vi "Eventos.vi"() -> ()   [LabVIEW 2018]
uses:
  <vilib>/RAFA Solutions/Harmony UI Controls Kit/String & Path/String Indicator.ctl
  <vilib>/RAFA Solutions/Harmony UI Controls Kit/Boolean/OK Button.ctl
  <vilib>/RAFA Solutions/Harmony UI Controls Kit/Boolean/Blank Button - Green.ctl
  Controls/Hora y Fecha control.ctl
  <vilib>/RAFA Solutions/Harmony UI Controls Kit/List, Table & Tree/Multicolumn Listbox.ctl
  <vilib>/RAFA Solutions/Harmony UI Controls Kit/Flat UI Design.lvlib
panel:
  in  "Tabla Eventos":T1
  out "fecha y hora":T2
  in  "Tiempo Final Eventos":timestamp caption="Tiempo Final" format="%<%X\n%x>T"
  in  "Tiempo Inicio Eventos":timestamp caption="Tiempo Inicio" format="%<%X\n%x>T"
  in  "Consultar Eventos":T3
  out "Generador":string
  in  "volver":T4
  out "Eventos":T5
  # "Sistema de Monitoreo de Calidad de Energía"
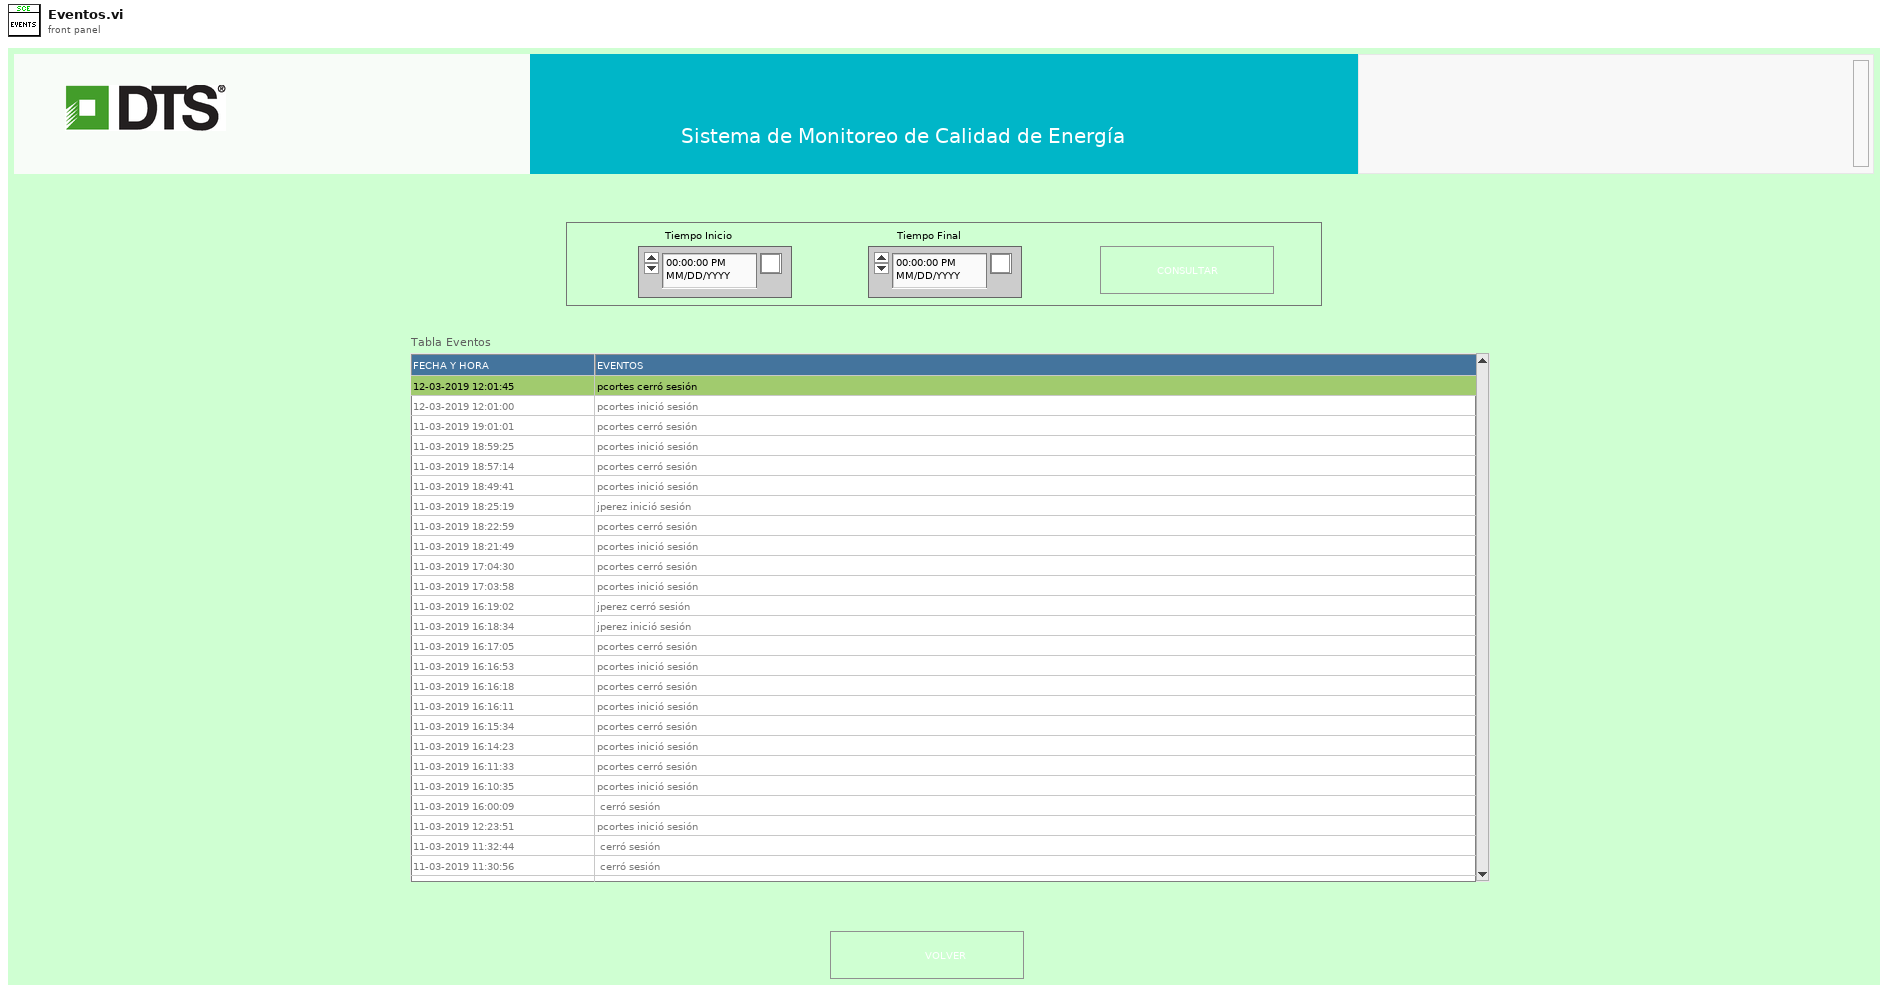
[diagram p1: front panel]
types:
  T1 = typedef "Flat UI Design.lvlib/Multicolumn Listbox.ctl" = i32
  T2 = typedef "Hora y Fecha control.ctl" = cluster{"fecha":string, "dia semana":string, "fecha 2":string}
  T3 = typedef "Flat UI Design.lvlib/Blank Button - Green.ctl" = bool
  T4 = typedef "Flat UI Design.lvlib/OK Button.ctl" = bool
  T5 = typedef "Flat UI Design.lvlib/String Indicator.ctl" = string
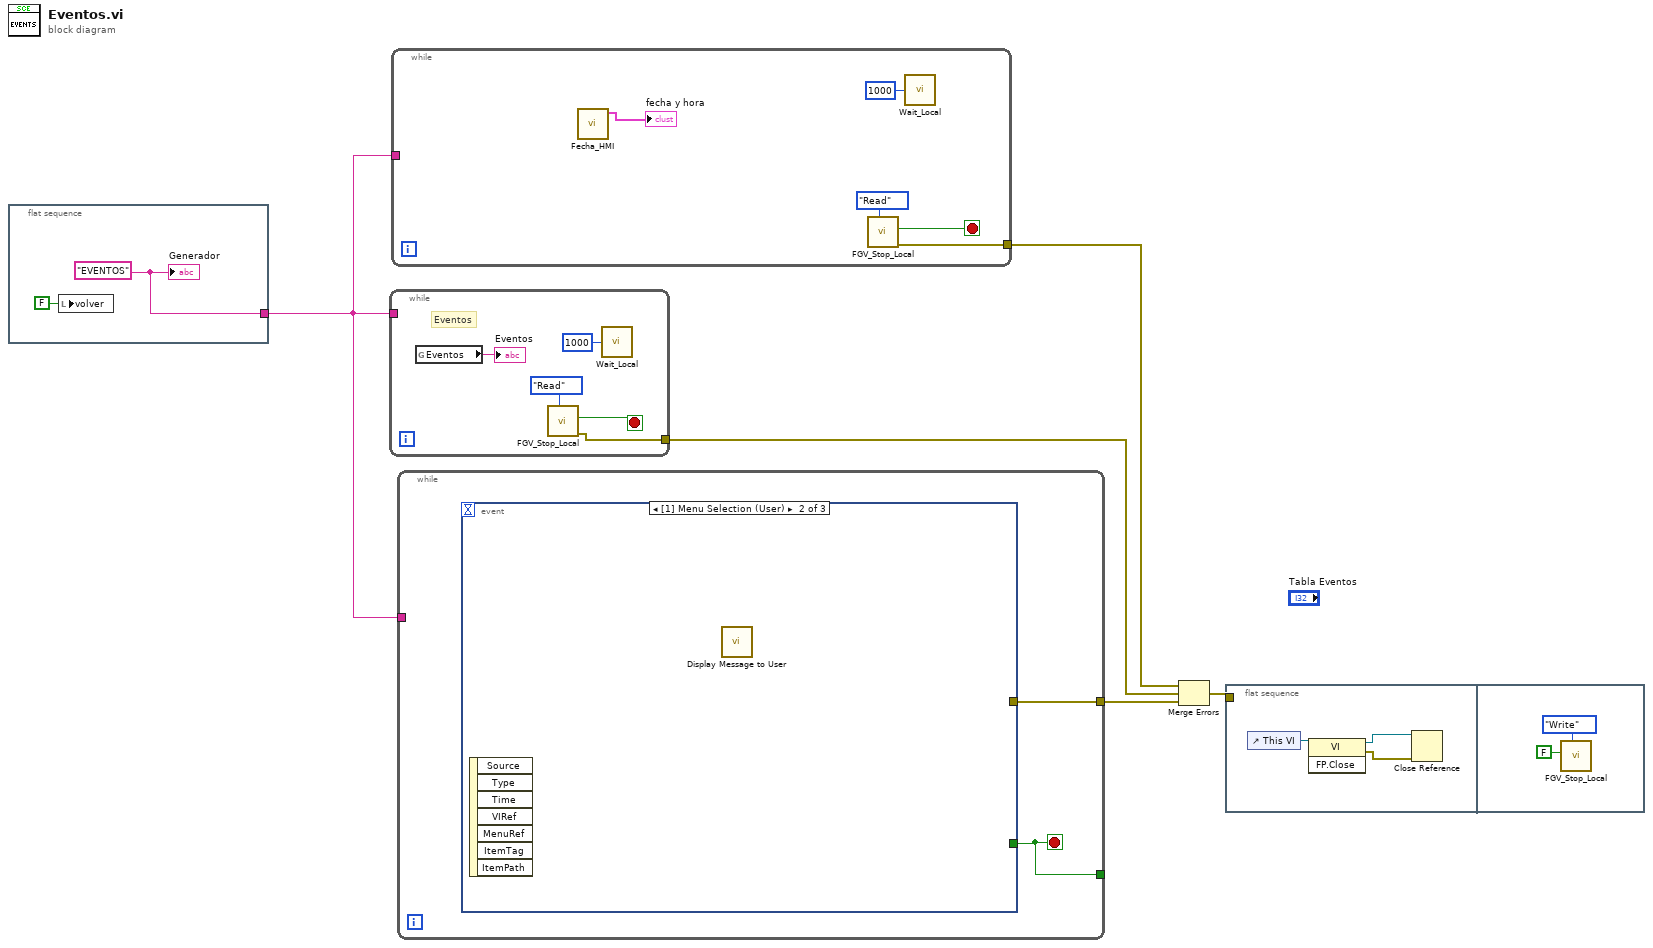
[diagram p0: block diagram]
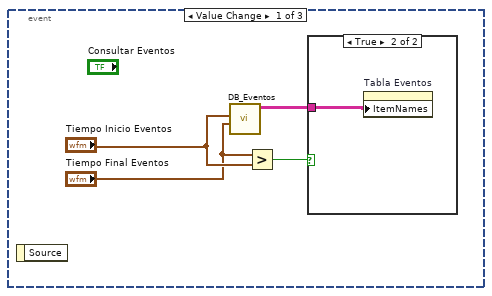
[diagram p2: hidden frame]
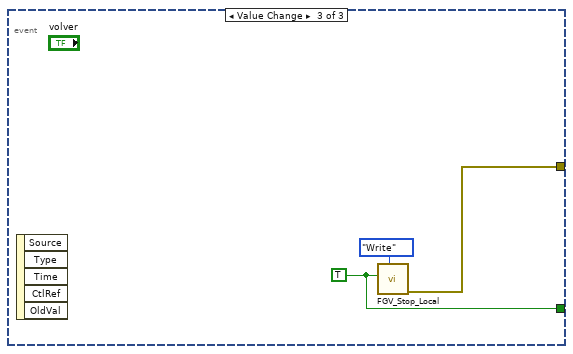
[diagram p4: hidden frame]
diagram:
  n1 = flat-sequence {
    tunnel: [w7] -> w5
    frame #0 {
      w7 = "EVENTOS" ("Generador in")
      n2 = local write "volver"(T4 FALSE ("volver")) -> ()
      "Generador" <- w7
    }
  }
  n3 = while {
    tunnel: w5 -> [_]
    tunnel: [w9] -> w4
    stop <- w11 stop-if-true
    # "Eventos"
    n4 = global read "globalEventos.vi" "Eventos"() -> (→"Eventos":string)
    n5 = call "FGV_Stop_Local.vi"("Action"=enum16{"Read", "Write"}."Read") -> ("Error Out"=w9:errorcluster, "Var Out"=w11:bool)  [unwired: 9 in]
    n6 = call "Wait_Local.vi"("Wait time (msec)"=u32 1000 ("milliseconds to wait")) -> ()  [unwired: 5 in]
  }
  n7 = while {
    tunnel: w5 -> [_]
    tunnel: [w14] -> w1
    stop <- w15 stop-if-true
    n8 = call "Fecha_HMI.vi"() -> ("fecha y hora"=→"fecha y hora":T2)  [unwired: 11 in]
    n9 = call "FGV_Stop_Local.vi"("Action"=enum16{"Read", "Write"}."Read") -> ("Error Out"=w14:errorcluster, "Var Out"=w15:bool)  [unwired: 9 in]
    n10 = call "Wait_Local.vi"("Wait time (msec)"=u32 1000 ("milliseconds to wait")) -> ()  [unwired: 5 in]
  }
  n11 = while {
    tunnel: w5 -> [_]
    tunnel: [w19] -> _
    tunnel: [w18] -> w3
    stop <- w19 stop-if-true
    n12 = event shown="[1] Menu Selection (User)" {
      selector: _ -> [_ _ _]
      dyn-events: _ -> [_ _ _]
      timeout: _ -> [_ _ _]
      tunnel: [_ _ w26] -> w19
      tunnel: [_ _ w25] -> w18
      event Value Change {
        n13 = event-data() -> ()  [unwired: 1 in, 1 out]
        n14 = call "DB_Eventos.vi"("Final"="Tiempo Final Eventos", "Inicio"="Tiempo Inicio Eventos") -> ("Data"=w23:string[][])  [unwired: 8 in, 1 out]
        n15 = Greater?(x="Tiempo Final Eventos", y="Tiempo Inicio Eventos") -> (0:w20:bool)
        n16 = case shown="True" w20 {
          tunnel: w23 -> [_ w24]
          frame False {
          }
          frame True {
            n17 = property on="Tabla Eventos" class="MCListbox (strict)"("ItemNames"=w24) -> ()  [unwired: 2 in, 2 out]
          }
        }
      }
      event Menu Selection (User) {
        n18 = event-data() -> ()  [unwired: 1 in, 7 out]
        n19 = call "Display Message to User"() -> ()  [unwired: 10 in, 2 out]
      }
      event Value Change {
        w26 = TRUE
        n20 = event-data() -> ()  [unwired: 1 in, 5 out]
        n21 = call "FGV_Stop_Local.vi"("Action"=enum16{"Read", "Write"}."Write", "Var In"=w26) -> ("Error Out"=w25:errorcluster)  [unwired: 8 in, 1 out]
      }
    }
  }
  n22 = Merge Errors(w1, w4, w3) -> (w2:errorcluster)
  n23 = flat-sequence {
    tunnel: w2 -> [_]
    frame #0 {
      n24 = control-ref of="This VI"() -> (w30:refnum<vi>)
      n25 = invoke class="VI" method="FP.Close"(reference=w30) -> (reference out=w29:refnum<vi>, error out=w28:errorcluster)  [unwired: 2 in, 1 out]
      n26 = Close Reference(reference=w29, error in (no error)=w28) -> ()  [unwired: 1 out]
    }
    frame #1 {
      n27 = call "FGV_Stop_Local.vi"("Action"=enum16{"Read", "Write"}."Write", "Var In"=FALSE) -> ()  [unwired: 8 in, 2 out]
    }
  }
